vi "IMUTilt.vi"(7 "Mag":T1, 9 "Accel":T2) -> (1 "Yaw":dbl(knob) scale=-180.0..180.0, 2 "Roll":dbl(knob) scale=-180.0..180.0, 3 "Pitch":dbl(knob) scale=-90.0..90.0)   [LabVIEW 2014]
doc: "Resets the gyroscope to a heading of zero. Use this VI to recalibrate the gyroscope after significant drift.\n\nThis software is licensed. Open the labview\\readme\\WPI Robotics Library Open Source License.txt file for more information."
uses:
  Accel.ctl
  Mag.ctl
panel:
  out "error":bool
  in  "tol":dbl=0.05
  # "When Sensor oriented with positive X-axis\npointing forward, and positive Y-axis\npointing left, and positive Z axis pointing up :\n\nRoll is rotation about X-axis, clockwise roll,\n(looking in + X direction), is positive.\n\nPitch is rotation about Y-axis, clockwise pitch\n(looking in + Y direction), is positive.\n\nYaw is rotation about Z-axis, clockwise yaw\n(looking in + Z direction), is positive."
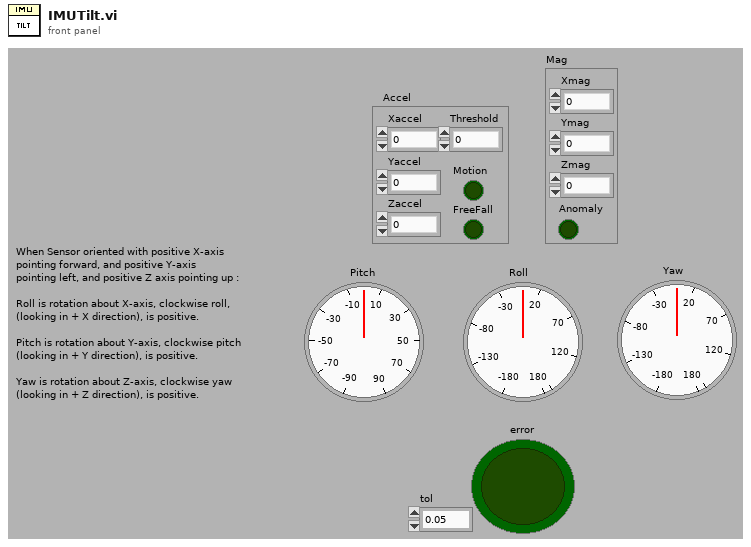
[diagram p1: front panel]
types:
  T1 = typedef "Mag.ctl" = cluster{"Xmag":dbl, "Ymag":dbl, "Zmag":dbl, "Anomaly":bool}
  T2 = typedef "Accel.ctl" = cluster{"Xaccel":dbl, "Yaccel":dbl, "Zaccel":dbl, "Motion":bool, "Threshold":dbl, "FreeFall":bool}
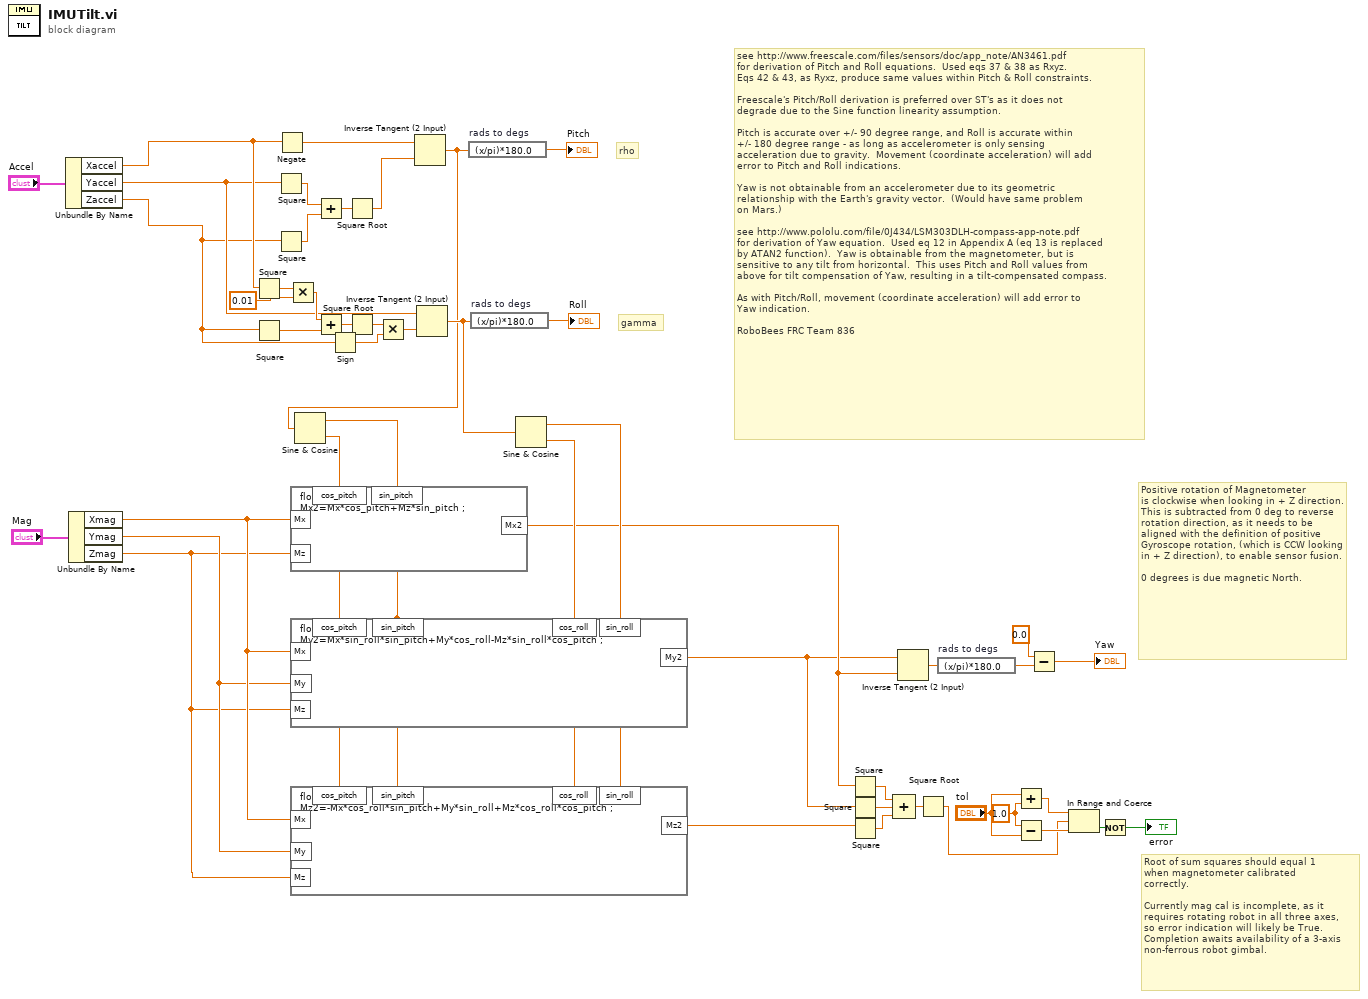
[diagram p0: block diagram]
diagram:
  w19 = 1.0 ("upper limit")
  # "Positive rotation of Magnetometer\nis clockwise when looking in + Z direction.  This is subtracted from 0 deg to reverse rotation direction, as it needs to be aligned with the definition of positive Gyroscope rotation, (which is CCW looking in + Z direction), to enable sensor fusion.\n\n0 degrees is due magnetic North."
  # "Root of sum squares should equal 1\nwhen magnetometer calibrated\ncorrectly.\n\nCurrently mag cal is incomplete, as it\nrequires rotating robot in all three axes, \nso error indication will likely be True.\nCompletion awaits availability of a 3-axis\nnon-ferrous robot gimbal."
  # "gamma"
  # "rho"
  # "see http://www.freescale.com/files/sensors/doc/app_note/AN3461.pdf\nfor derivation of Pitch and Roll equations.  Used eqs 37 & 38 as Rxyz.\nEqs 42 & 43, as Ryxz, produce same values within Pitch & Roll constraints.\n\nFreescale's Pitch/Roll derivation is preferred over ST's as it does not\ndegrade due to the Sine function linearity assumption.\n\nPitch is accurate over +/- 90 degree range, and Roll is accurate within\n+/- 180 degree range - as long as accelerometer is only sensing\nacceleration due to gravity.  Movement (coordinate acceleration) will add\nerror to Pitch and Roll indications.\n\nYaw is not obtainable from an accelerometer due to its geometric \nrelationship with the Earth's gravity vector.  (Would have same problem\non Mars.)\n\nsee http://www.pololu.com/file/0J434/LSM303DLH-compass-app-note.pdf\nfor derivation of Yaw equation.  Used eq 12 in Appendix A (eq 13 is replaced\nby ATAN2 function).  Yaw is obtainable from the magnetometer, but is\nsensitive to any tilt from horizontal.  This uses Pitch and Roll values from\nabove for tilt compensation of Yaw, resulting in a tilt-compensated compass.\n\nAs with Pitch/Roll, movement (coordinate acceleration) will add error to\nYaw indication.\n\nRoboBees FRC Team 836"
  n1 = Unbundle By Name("Accel") -> ("Xaccel"=w34:dbl, "Yaccel"=w33:dbl, "Zaccel"=w32:dbl)
  n2 = Unbundle By Name("Mag") -> ("Xmag"=w11:dbl, "Ymag"=w10:dbl, "Zmag"=w9:dbl)
  n3 = Square(x=w34) -> (x^2=w42:dbl)
  n4 = Square(x=w32) -> (x^2=w39:dbl)
  n5 = Square(x=w33) -> (x^2=w35:dbl)
  n6 = Square(x=w32) -> (x^2=w36:dbl)
  n7 = Negate(x=w34) -> (-x=w44:dbl)
  n8 = Multiply(x=w42, y=0.01 ("u 2")) -> (x*y=w43:dbl)
  n9 = Add(x=w35, y=w36) -> (x+y=w37:dbl)
  n10 = Add(x=w43, y=w39) -> (x+y=w38:dbl)
  n11 = Sign(1:w32) -> (0:w41:dbl)
  n12 = Square Root(x=w37) -> (sqrt(x)=w45:dbl)
  n13 = Square Root(x=w38) -> (sqrt(x)=w40:dbl)
  n14 = Multiply(x=w40, y=w41) -> (x*y=w46:dbl)
  n15 = Inverse Tangent (2 Input)(1:w45, 2:w44) -> (0:w2:dbl)
  n16 = Sine & Cosine(0:w2) -> (1:w28:dbl, 2:w29:dbl)
  n17 = formula code="float Mx2;\nMx2=Mx*cos_pitch+Mz*sin_pitch ;"("Mx"=w11, "cos_pitch"=w29, "sin_pitch"=w28, "Mz"=w9) -> ("Mx2"=w13:dbl)
  n18 = Inverse Tangent (2 Input)(1:w46, 2:w33) -> (0:w3:dbl)
  n19 = expression code="(x/pi)*180.0" "rads to degs"(w2) -> (→"Pitch":dbl)
  n20 = expression code="(x/pi)*180.0" "rads to degs"(w3) -> (→"Roll":dbl)
  n21 = Sine & Cosine(0:w3) -> (1:w26:dbl, 2:w27:dbl)
  n22 = formula code="float My2;\nMy2=Mx*sin_roll*sin_pitch+My*cos_roll-Mz*sin_roll*cos_pitch ;"("Mx"=w11, "cos_pitch"=w29, "sin_pitch"=w28, "Mz"=w9, "My"=w10, "sin_roll"=w26, "cos_roll"=w27) -> ("My2"=w12:dbl)
  n23 = formula code="float Mz2;\nMz2=-Mx*cos_roll*sin_pitch+My*sin_roll+Mz*cos_roll*cos_pitch ;"("Mx"=w11, "cos_pitch"=w29, "sin_pitch"=w28, "Mz"=w9, "My"=w10, "sin_roll"=w26, "cos_roll"=w27) -> ("Mz2"=w22:dbl)
  n24 = Square(x=w13) -> (x^2=w21:dbl)
  n25 = Square(x=w12) -> (x^2=w25:dbl)
  n26 = Square(x=w22) -> (x^2=w24:dbl)
  n27 = Compound Arithmetic op=ADD(w21, w25, w24) -> (w23:dbl)
  n28 = Inverse Tangent (2 Input)(1:w13, 2:w12) -> (0:w6:dbl)
  n29 = Square Root(x=w23) -> (sqrt(x)=w16:dbl)
  n30 = expression code="(x/pi)*180.0" "rads to degs"(w6) -> (w5:dbl)
  n31 = Add(x="tol", y=w19) -> (x+y=w20:dbl)
  n32 = Subtract(x=w19, y="tol") -> (x-y=w18:dbl)
  n33 = Subtract(x=0.0, y=w5) -> (x-y=→"Yaw":dbl)
  n34 = In Range and Coerce(upper limit=w20, x=w16, lower limit=w18) -> (In Range?=w17:bool)  [unwired: 1 out]
  n35 = Not(x=w17) -> (.not. x?=→"error":bool)
